vi "Get SubNumber.vi"(8 "error in":errorcluster, 11 "DOMAIN in":refnum<class "DOMAIN.lvclass">) -> (0 "error out":errorcluster, 1 "Defined?":bool, 2 "SubNumber":u8 format="%.0x", 3 "DOMAIN out":refnum<class "DOMAIN.lvclass">)   [LabVIEW 2019, in "Electronic Datasheet.lvlib" / "DOMAIN.lvclass"]
uses:
  DOMAIN.lvclass
  Electronic Datasheet.lvlib
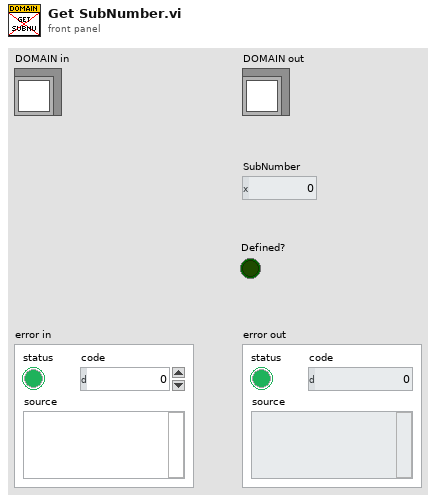
[diagram p1: front panel]
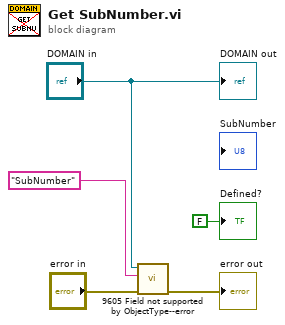
[diagram p0: block diagram]
diagram:
  n1 = call "9605 Field not supported by ObjectType--error.vi"("error in"="error in", "Field Name"="SubNumber" ("Field name"), "Object Type Base"="DOMAIN in") -> ("error out"=→"error out":errorcluster)  [unwired: 7 in, 1 out]
  "DOMAIN out" <- "DOMAIN in"
  "Defined?" <- FALSE ("Set?")
